vi "Find First Matched Pattern.vi"(9 "Numeric in":i32, 10 "RE characters to match (must be pre-escaped)":string[](array[string]), 11 "trimmed string in":string) -> (1 "offset past match":i32, 2 "match":string)   [LabVIEW 2020, in "jki_python_data_tools.lvlib"]
uses:
  jki_python_data_tools.lvlib
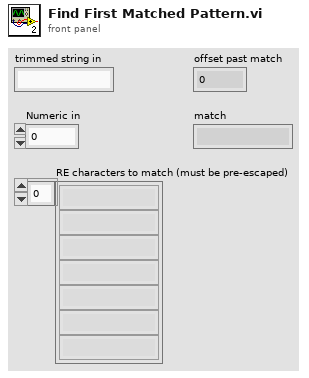
[diagram p1: front panel]
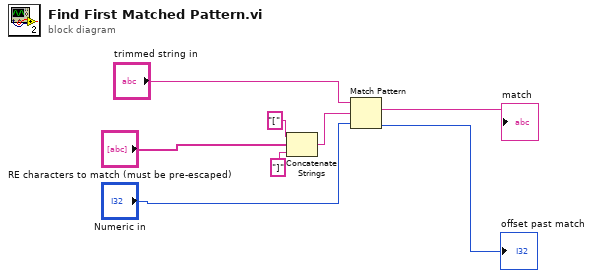
[diagram p0: block diagram]
diagram:
  n1 = Concatenate Strings("[" ("string"), "RE characters to match (must be pre-escaped)", "]" ("string")) -> (w2:string)
  n2 = Match Pattern(string="trimmed string in", regular expression=w2, offset (0)="Numeric in") -> (match substring=→"match":string, offset past match=→"offset past match":i32)  [unwired: 2 out]
